vi "WPI_IMU_Loop.vi"(8 "error in":errorcluster, 11 "ADI IMU Interrupt DevRef":T1={"SimpleGyroDevRef"={"DevStatus"={"status"=FALSE, "code"=0, "source"=""}, "Handle"=0, "SPI Bus"=enum."SPI On-Board, CS0", "Device Found"=FALSE, "Sample Rate"=0.0, "Device Ready"=FALSE, "Yaw Axis"=enum."Z", "AHRS Algorithm"=enum."Complementary"}, "InterruptRef"={"DevStatus"={"status"=FALSE, "code"=0, "source"=""}, "InterruptIndex"=enum."0"}} {"SimpleGyroDevRef"."Sample Rate" min=0.25 max=100.0 step=0.25}) -> (0 "error out":errorcluster, 1 "Device Found":bool)   [LabVIEW 2015, in "FRC ADI MXP IMU.lvlib"]
doc: "Periodically reads the ADI MXP IMU valuse and makes data available for use elsewhere in your robot project. Place this block within PeriodicTasks.vi outside any loops."
uses:
  FRC ADI MXP IMU.lvlib
  WPI_AnalogDevicesIMUInterruptDevRef.ctl
  WPI_AnalogDevicesIMUDevRef.ctl
  <vilib>/Rock Robotics/SystemInterfaces/spilib/spi_bus.ctl
  <vilib>/Rock Robotics/WPI/Interrupt/WPI_InterruptRef.ctl
  <vilib>/Rock Robotics/SystemInterfaces/Interrupt/FPGA_InterruptIndex.ctl
  <vilib>/Rock Robotics/WPI/SPI/WPI_SPIDevRef.ctl
  <vilib>/Platform/TimedLoop/XDataNode/timing_clust.ctl
  <vilib>/Platform/TimedLoop/XDataNode/nitl_modes.ctl
  <vilib>/Platform/TimedLoop/XDataNode/wakeup.ctl
  <vilib>/Rock Robotics/SystemInterfaces/Interrupt/FPGA_WaitOnInterrupt.vi
  <vilib>/Rock Robotics/WPI/Utilities/WPI_UtilitiesTimebaseConstants.vi
  <vilib>/Rock Robotics/SystemInterfaces/Interrupt/FPGA_InterruptReadTimestamp.vi
  <vilib>/platform/TimedLoop/XDataNode/XDataNode.xnode
  <vilib>/ptbypt/NI_PtbyPt.lvlib
  <vilib>/Platform/TimedLoop/XDataNode/XDNodeRunTimeDep.lvlib
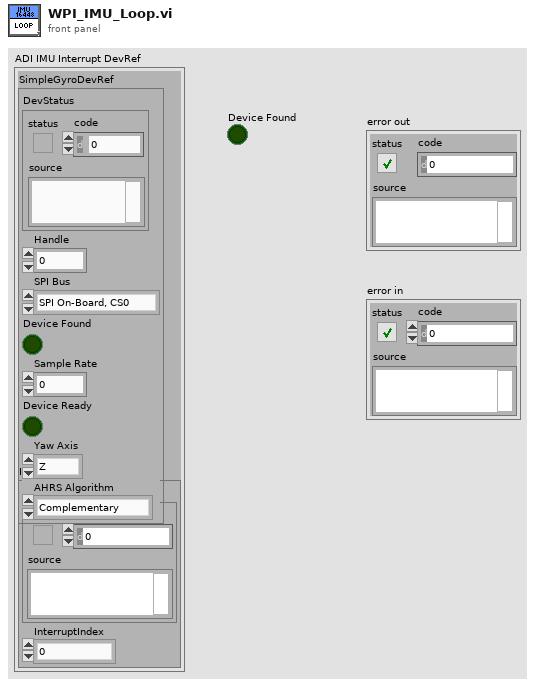
[diagram p1: front panel]
types:
  T1 = typedef "FRC ADI MXP IMU.lvlib/WPI_AnalogDevicesIMUInterruptDevRef.ctl" = cluster{"SimpleGyroDevRef":T2, "InterruptRef":T4}
  T2 = typedef "FRC ADI MXP IMU.lvlib/WPI_AnalogDevicesIMUDevRef.ctl" = cluster{"DevStatus":errorcluster, "Handle":i32, "SPI Bus":T3, "Device Found":bool, "Sample Rate":dbl, "Device Ready":bool, "Yaw Axis":enum16{"X", "Y", "Z"}, "AHRS Algorithm":enum16{"Complementary", "Madgwick"}}
  T3 = typedef "spi_bus.ctl" = enum16{"SPI On-Board, CS0", "SPI On-Board, CS1", "SPI On-Board, CS2", "SPI On-Board, CS3", "SPI MXP", "Invalid"}
  T4 = typedef "WPI_InterruptRef.ctl" = cluster{"DevStatus":errorcluster, "InterruptIndex":T5}
  T5 = typedef "FPGA_InterruptIndex.ctl" = enum8{"0", "1", "2", "3", "4", "5", "6", "7", "Invalid"}
  T6 = typedef "WPI_SPIDevRef.ctl" = cluster{"DevStatus":errorcluster, "Handle":i32, "SPI Bus":T3}
  T7 = cluster{"X Crossover":dbl, "Y Crossover":dbl, "Z Crossover":dbl, "X Range":dbl, "Y Range":dbl, "Z Range":dbl, "X Angle":dbl, "Y Angle":dbl, "Z Angle":dbl}
  T8 = cluster{"Output[0]":dbl, "Output[1]":dbl, "Output[2]":dbl}
  T9 = typedef "XDNodeRunTimeDep.lvlib/timing_clust.ctl" = cluster{"Expected End [f-1]":u64, "Actual End [f-1]":u64, "Finished Late? [f-1]":bool, "Expected End [i-1]":u64, "Actual End [i-1]":u64, "Finished Late? [i-1]":bool, "Expected Start [i]":u64, "Actual Start [i]":u64, "Expected Start [f]":u64, "Actual Start [f]":u64, "Source Name":string, "Structure Name":string, "Period":i64, "Deadline":i64, "Offset":i64, "Start":i64, "Priority":i32, "Timeout":i32, "Mode":T10, "Wakeup Reason":T11, "Error":errorcluster, "Source Type":string, "Secondary Source Type":string, "Global End Time":u64, "Global Start Time":u64, "Frame Duration":u64, "Iteration Duration":u64, "Assigned CPU":i32, "I/O Scan Engine Mode":u32}
  T10 = typedef "XDNodeRunTimeDep.lvlib/nitl_modes.ctl" = enum32{"No Change", "Process missed periods, maintain original phase", "Discard missed periods, maintain original phase", "Process missed periods, ignore original phase", "Discard missed periods, ignore original phase"}
  T11 = typedef "XDNodeRunTimeDep.lvlib/wakeup.ctl" = enum32{"Normal", "Aborted", "Asynchronous wakeup", "Timing source error", "Timed loop error", "Timeout"}
  T12 = cluster{"Data Array[0]":dbl, "Data Array[1]":dbl, "Data Array[2]":dbl, "Data Array[3]":dbl, "Data Array[4]":dbl, "Data Array[5]":dbl, "Data Array[6]":dbl, "Data Array[7]":dbl, "Data Array[8]":dbl, "Data Array[9]":dbl, "Data Array[10]":dbl}
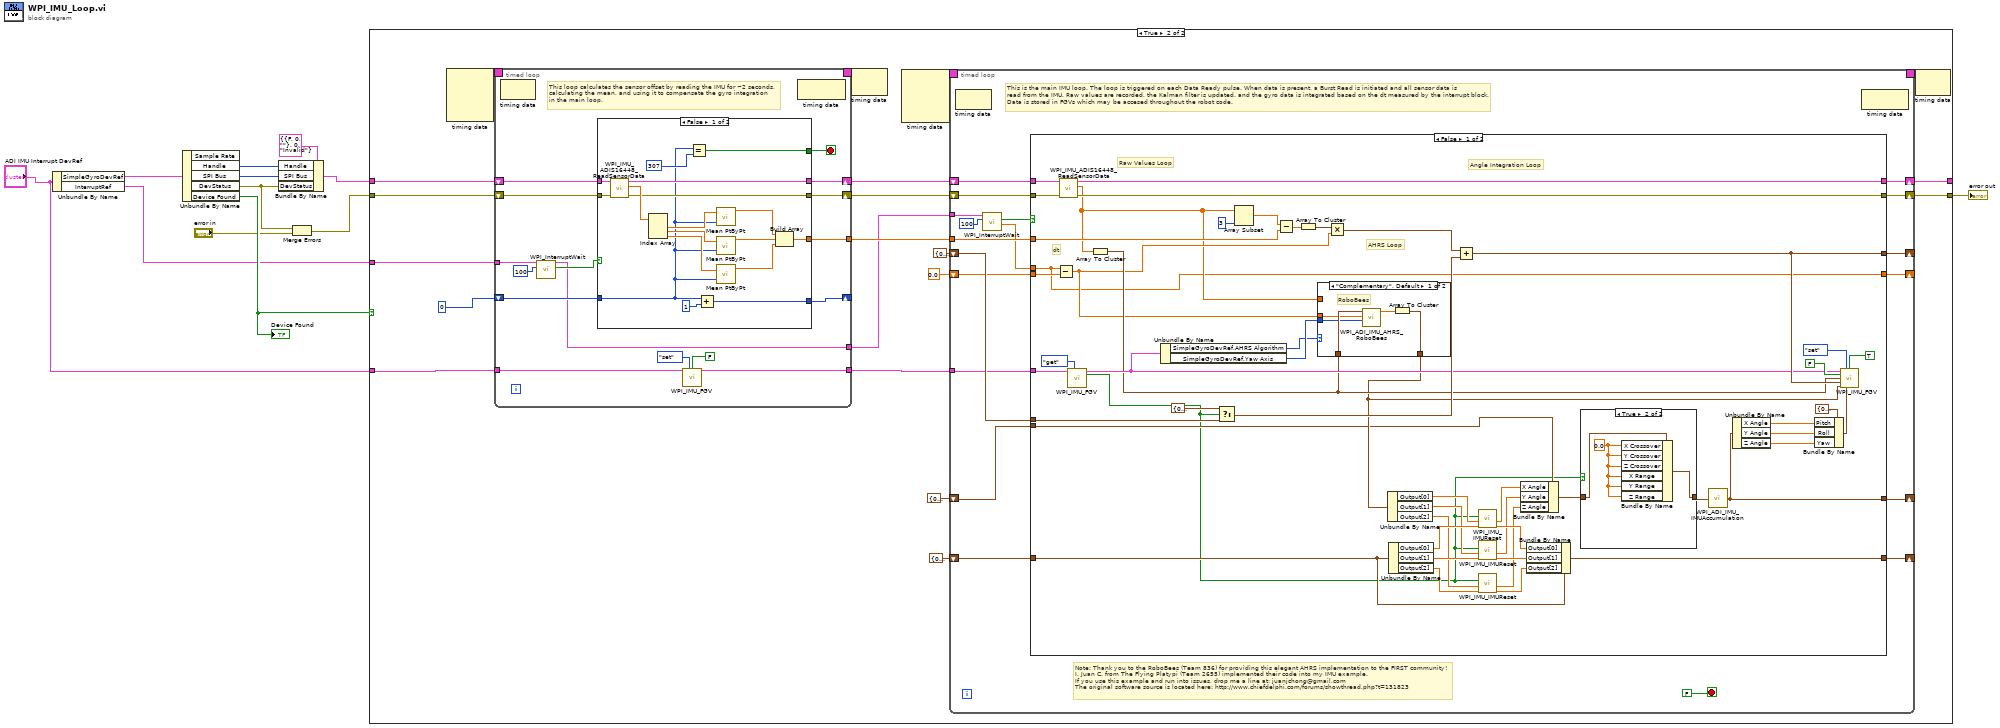
[diagram p0: block diagram]
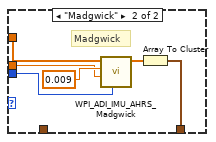
[diagram p4: hidden frame]
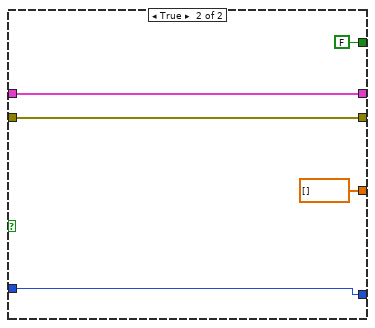
[diagram p6: hidden frame]
diagram:
  n1 = Unbundle By Name("ADI IMU Interrupt DevRef") -> ("SimpleGyroDevRef"=w6:T2, "InterruptRef"=w5:T4)
  n2 = Unbundle By Name(w6) -> ("Handle"=w11:i32, "SPI Bus"=w10:T3, "DevStatus"=w3:errorcluster, "Device Found"=w9:bool)  [unwired: 1 out]
  "Device Found" <- w9
  n3 = Bundle By Name(cluster=T6 {"DevStatus"={"status"=FALSE, "code"=0, "source"=""}, "Handle"=0, "SPI Bus"=enum."Invalid"} ("SPIDevRef out"), "Handle"=w11, "SPI Bus"=w10, "DevStatus"=w3) -> (w8:T6)
  n4 = Merge Errors(w3, "error in") -> (w1:errorcluster)
  n5 = case shown="True" w9 {
    tunnel: w8 -> [w14 w32]
    tunnel: w1 -> [w13 w31]
    tunnel: [w13 w34] -> w7
    tunnel: [w14 w33] -> _
    tunnel: "ADI IMU Interrupt DevRef" -> [_ w19]
    tunnel: w5 -> [_ w21]
    frame False {
    }
    frame True {
      n6 = node-c288() -> (w23:T9)  [unwired: 4 in]
      n7 = timed-loop {
        tunnel: [w143] -> w27
        shift-right: [w145] -> w29
        shift-left: w32 -> [w137]
        shift-right: [w146] -> w30
        shift-left: w31 -> [w136]
        shift-right: [w141] -> _
        shift-left: 0 -> [w142]
        tunnel: w21 -> [w140]
        tunnel: [w135] -> w25
        timing: w23 -> [_]
        timing-out: [_] -> w22
        tunnel: w19 -> [w133]
        tunnel: [w134] -> w16
        stop <- w144 stop-if-true
        # "This loop calculates the sensor offset by reading the IMU for ~2 seconds, \ncalculating the mean, and using it to compensate the gyro integration\nin the main loop."
        n8 = node-c288() -> ()  [unwired: 1 in, 1 out]
        n9 = call <vilib>:"WPI_InterruptWait.vi"("Timeout (ms)"=100, "InterruptRef"=w140) -> ("Timed Out"=w138:bool, "InterruptRef"=w135:T4)  [unwired: 5 in, 3 out]
        n10 = case shown="False" w138 {
          tunnel: [w164 w167] -> w146
          tunnel: [w163 w168] -> w145
          tunnel: [w158 FALSE] -> w144
          tunnel: [w154 dbl[] []] -> w143
          tunnel: w136 -> [w153 w167]
          tunnel: w137 -> [w152 w168]
          tunnel: w142 -> [w149 w170]
          tunnel: [w151 w170] -> w141
          frame False {
            n11 = call "WPI_IMU_ADIS16448_ReadSensorData.vi"("error in (no error)"=w153, "SPIDevRef in"=w152) -> ("error out"=w164:errorcluster, "Data Array"=w165:dbl[], "SPIDevRef out"=w163:T6)  [unwired: 7 in]
            n12 = Index Array(array=w165) -> (element #1=w162:dbl, element #2=w161:dbl, element #3=w160:dbl)  [unwired: 3 in]
            n13 = Equal?(x=w149, y=307) -> (x = y?=w158:bool)
            n14 = Add(x=w149, y=1) -> (x+y=w151:i32)
            n15 = call <vilib>:"Mean PtByPt.vi"("x"=w162, "sample length"=w149) -> ("mean"=w157:dbl)  [unwired: 2 in, 1 out]
            n16 = call <vilib>:"Mean PtByPt.vi"("x"=w161, "sample length"=w149) -> ("mean"=w156:dbl)  [unwired: 2 in, 1 out]
            n17 = call <vilib>:"Mean PtByPt.vi"("x"=w160, "sample length"=w149) -> ("mean"=w155:dbl)  [unwired: 2 in, 1 out]
            n18 = Build Array(w157, w156, w155) -> (w154:dbl[])
          }
          frame True {
          }
        }
        n19 = call "WPI_IMU_FGV.vi"("ADI IMU Interrupt DevRef"=w133, "Operation"=enum16{"set", "get"}."set", "Sensor Ready?"=FALSE) -> ("ADI IMU Interrupt DevRef Out"=w134:T1)  [unwired: 6 in, 6 out]
        n20 = node-c288() -> ()  [unwired: 1 in, 1 out]
      }
      n21 = node-c288(w22) -> ()  [unwired: 1 out]
      n22 = node-c288() -> (w18:T9)  [unwired: 4 in]
      n23 = timed-loop {
        shift-right: [w53] -> w33
        shift-left: w29 -> [w47]
        shift-right: [w52] -> w34
        shift-left: w30 -> [w46]
        shift-right: [w50] -> _
        shift-left: cluster{dbl, dbl, dbl} {0.0, 0.0, 0.0} -> [w49]
        tunnel: w27 -> [w48]
        tunnel: w25 -> [w44]
        shift-right: [w37] -> _
        shift-left: 0.0 ("TimeStamp") -> [w42]
        shift-right: [w39] -> _
        shift-left: T8 {"Output[0]"=0.0, "Output[1]"=0.0, "Output[2]"=0.0} -> [w41]
        tunnel: w16 -> [w38]
        timing: w18 -> [_]
        timing-out: [_] -> w17
        shift-right: [w36] -> _
        shift-left: T7 {"X Crossover"=0.0, "Y Crossover"=0.0, "Z Crossover"=0.0, "X Range"=0.0, "Y Range"=0.0, "Z Range"=0.0, "X Angle"=0.0, "Y Angle"=0.0, "Z Angle"=0.0} ("Input Data") -> [w35]
        stop <- FALSE stop-if-true
        # "Note: Thank you to the RoboBees (Team 836) for providing this elegant AHRS implementation to the FIRST community!\nI, Juan C. from The Flying Platypi (Team 2655) implemented their code into my IMU example.\nIf you use this example and run into issues, drop me a line at: juanjchong@gmail.com\nThe original software source is located here: http://www.chiefdelphi.com/forums/showthread.php?t=131823"
        # "This is the main IMU loop. The loop is triggered on each Data Ready pulse. When data is present, a Burst Read is initiated and all sensor data is \nread from the IMU. Raw values are recorded, the Kalman filter is updated, and the gyro data is integrated based on the dt measured by the interrupt block.\nData is stored in FGVs which may be accesed throughout the robot code."
        n24 = node-c288() -> ()  [unwired: 1 in, 1 out]
        n25 = call <vilib>:"WPI_InterruptWait.vi"("Timeout (ms)"=100, "InterruptRef"=w44) -> ("TimeStamp"=w43:dbl, "Timed Out"=w40:bool)  [unwired: 5 in, 3 out]
        n26 = case shown="False" w40 {
          tunnel: w47 -> [w107 w128]
          tunnel: w46 -> [w106 w127]
          tunnel: [w105 w128] -> w53
          tunnel: [w104 w127] -> w52
          tunnel: w38 -> [w89 _]
          tunnel: [w97 w126] -> w50
          tunnel: w49 -> [w100 w126]
          tunnel: w48 -> [w95 _]
          tunnel: w43 -> [w81 _]
          tunnel: w42 -> [w91 w124]
          tunnel: w41 -> [w71 w125]
          tunnel: [w68 w125] -> w39
          tunnel: [w81 w124] -> w37
          tunnel: [w59 w123] -> w36
          tunnel: w35 -> [w69 w123]
          frame False {
            # "dt"
            # "Angle Integration Loop"
            # "AHRS Loop"
            # "Raw Values Loop"
            n27 = Subtract(x=w81, y=w91) -> (x-y=w85:dbl)
            n28 = call "WPI_IMU_ADIS16448_ReadSensorData.vi"("error in (no error)"=w106, "SPIDevRef in"=w107) -> ("error out"=w104:errorcluster, "Data Array"=w83:dbl[], "SPIDevRef out"=w105:T6)  [unwired: 7 in]
            n29 = call "WPI_IMU_FGV.vi"("ADI IMU Interrupt DevRef"=w89, "Operation"=enum16{"set", "get"}."get") -> ("ADI IMU Interrupt DevRef Out"=w87:T1, "Reset Out"=w62:bool)  [unwired: 7 in, 5 out]
            n30 = Array To Cluster(array=w83) -> (cluster=w86:T12)
            n31 = Unbundle By Name(w87) -> ("SimpleGyroDevRef.AHRS Algorithm"=w82:enum16{"Complementary", "Madgwick"}, "SimpleGyroDevRef.Yaw Axis"=w84:enum16{"X", "Y", "Z"})
            n32 = Select(t=T8 {"Output[0]"=0.0, "Output[1]"=0.0, "Output[2]"=0.0} ("cluster"), s=w62, f=w100) -> (s? t:f=w99:T8)
            n33 = Array Subset(array=w83, length=3) -> (w96:dbl[])  [unwired: 1 in]
            n34 = Subtract(x=w96, y=w95) -> (x-y=w94:dbl[])
            n35 = Array To Cluster(array=w94) -> (cluster=w93:cluster{"[0]":dbl, "[1]":dbl, "[2]":dbl})
            n36 = case shown="\"Complementary\", Default" w82 {
              tunnel: [w115 w120] -> w70
              tunnel: w86 -> [w114 _]
              tunnel: w85 -> [w113 w119]
              tunnel: w84 -> [w112 w117]
              tunnel: w83 -> [_ w118]
              frame "Complementary", Default {
                # "RoboBees"
                n37 = call "WPI_ADI_IMU_AHRS_RoboBees.vi"("Yaw Axis"=w112, "dt (s)"=w113, "IMU Rates"=w114) -> ("Output"=w116:dbl[])  [unwired: 4 in, 3 out]
                n38 = Array To Cluster(array=w116) -> (cluster=w115:T8)
              }
              frame "Madgwick" {
                # "Madgwick"
                n39 = call "WPI_ADI_IMU_AHRS_Madgwick.vi"("Yaw Axis"=w117, "dt (s)"=w119, "Beta"=0.009, "Data"=w118) -> ("Output"=w121:dbl[])  [unwired: 7 in]
                n40 = Array To Cluster(array=w121) -> (cluster=w120:T8)
              }
            }
            n41 = Multiply(x=w93, y=w85) -> (x*y=w92:cluster{"[0]":dbl, "[1]":dbl, "[2]":dbl})
            n42 = Unbundle By Name(w70) -> ("Output[0]"=w77:dbl, "Output[1]"=w76:dbl, "Output[2]"=w75:dbl)
            n43 = Unbundle By Name(w71) -> ("Output[0]"=w80:dbl, "Output[1]"=w79:dbl, "Output[2]"=w78:dbl)
            n44 = Add(x=w92, y=w99) -> (x+y=w97:cluster{dbl, dbl, dbl})
            n45 = call "WPI_IMU_IMUReset.vi"("AHRS Reset In"=w80, "Absolute Angle"=w77, "Reset"=w62) -> ("AHRS Reset Out"=w74:dbl, "Converted Output"=w67:dbl)  [unwired: 5 in]
            n46 = call "WPI_IMU_IMUReset.vi"("AHRS Reset In"=w79, "Absolute Angle"=w76, "Reset"=w62) -> ("AHRS Reset Out"=w73:dbl, "Converted Output"=w66:dbl)  [unwired: 5 in]
            n47 = call "WPI_IMU_IMUReset.vi"("AHRS Reset In"=w78, "Absolute Angle"=w75, "Reset"=w62) -> ("AHRS Reset Out"=w72:dbl, "Converted Output"=w65:dbl)  [unwired: 5 in]
            n48 = Bundle By Name(cluster=w69, "X Angle"=w67, "Y Angle"=w66, "Z Angle"=w65) -> (w63:T7)
            n49 = Bundle By Name(cluster=w71, "Output[0]"=w74, "Output[1]"=w73, "Output[2]"=w72) -> (w68:T8)
            n50 = case shown="True" w62 {
              tunnel: [w108 w110] -> w64
              tunnel: w63 -> [w108 w111]
              frame False {
              }
              frame True {
                w109 = 0.0
                n51 = Bundle By Name(cluster=w111, "X Crossover"=w109, "Y Crossover"=w109, "Z Crossover"=w109, "X Range"=w109, "Y Range"=w109, "Z Range"=w109) -> (w110:T7)
              }
            }
            n52 = call "WPI_ADI_IMU_IMUAccumulation.vi"("Input Data"=w64) -> ("Output Data"=w59:T7)
            n53 = Unbundle By Name(w59) -> ("X Angle"=w58:dbl, "Y Angle"=w57:dbl, "Z Angle"=w56:dbl)
            n54 = Bundle By Name(cluster=cluster{"Pitch":dbl, "Roll":dbl, "Yaw":dbl} {"Pitch"=0.0, "Roll"=0.0, "Yaw"=0.0} ("IMU AHRS DELTA"), "Pitch"=w58, "Roll"=w57, "Yaw"=w56) -> (w60:cluster{"Pitch":dbl, "Roll":dbl, "Yaw":dbl})
            n55 = call "WPI_IMU_FGV.vi"("ADI IMU Interrupt DevRef"=w87, "Operation"=enum16{"set", "get"}."set", "Sensor Ready?"=TRUE, "Reset"=FALSE ("Calibrated"), "IMU Data"=w86, "IMU Angles"=w97, "IMU AHRS"=w70, "IMU AHRS DELTA"=w60) -> ()  [unwired: 1 in, 7 out]
          }
          frame True {
            # "Waiting for an interrupt..."
          }
        }
        n56 = node-c288() -> ()  [unwired: 1 in, 1 out]
      }
      n57 = node-c288(w17) -> ()  [unwired: 1 out]
    }
  }
  "error out" <- w7
